vi "AxisControl.vi"(0 "String in":string, 1 "AxisBounds":T5={"Min"={"Auto"=TRUE, "Value"=0.0}, "Max"={"Auto"=TRUE, "Value"=0.0}}, 3 "ticsAndGrids":T2={"tics"={"Auto"=FALSE, "ticMin"=0.0, "ticStep"=0.0, "ticMax"=0.0, "minorDivsPerMajor"=0, "Mirror tics"=TRUE}, "Grids"={"Gridlines"=enum."No grids", "Zeroaxis"=enum."No zero axis"}}, 5 "Axis":T7="x", 9 "ShowNumbers?":bool=TRUE, 11 "ShowLabel?":bool=TRUE, 12 "Axis Label":string, 13 "Min tic value":dbl=0.001, 14 "Values":dbl[](array[numeric]), 15 "No of Tics":i32=2) -> (4 "String out":string)   [LabVIEW 2012]
uses:
  axisName.ctl
  minAndMax.ctl
  AxisScale.ctl
  ticsAndGrids.ctl
  tics.ctl
  grids.ctl
  commandArray.ctl
panel:
  out "Commands":T1
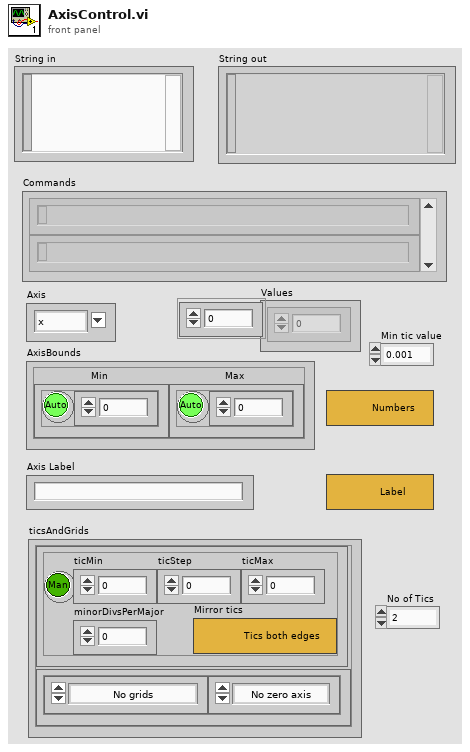
[diagram p1: front panel]
types:
  T1 = typedef "commandArray.ctl" = string[]
  T2 = typedef "ticsAndGrids.ctl" = cluster{"tics":T3, "Grids":T4}
  T3 = typedef "tics.ctl" = cluster{"Auto":bool, "ticMin":dbl, "ticStep":dbl, "ticMax":dbl, "minorDivsPerMajor":i32, "Mirror tics":bool}
  T4 = typedef "grids.ctl" = cluster{"Gridlines":enum16{"No grids", "Major grid", "Minor grid", "Major and Minor"}, "Zeroaxis":enum16{"No zero axis", "Show zero axis"}}
  T5 = typedef "minAndMax.ctl" = cluster{"Min":T6, "Max":T6}
  T6 = typedef "AxisScale.ctl" = cluster{"Auto":bool, "Value":dbl}
  T7 = typedef "axisName.ctl" = string
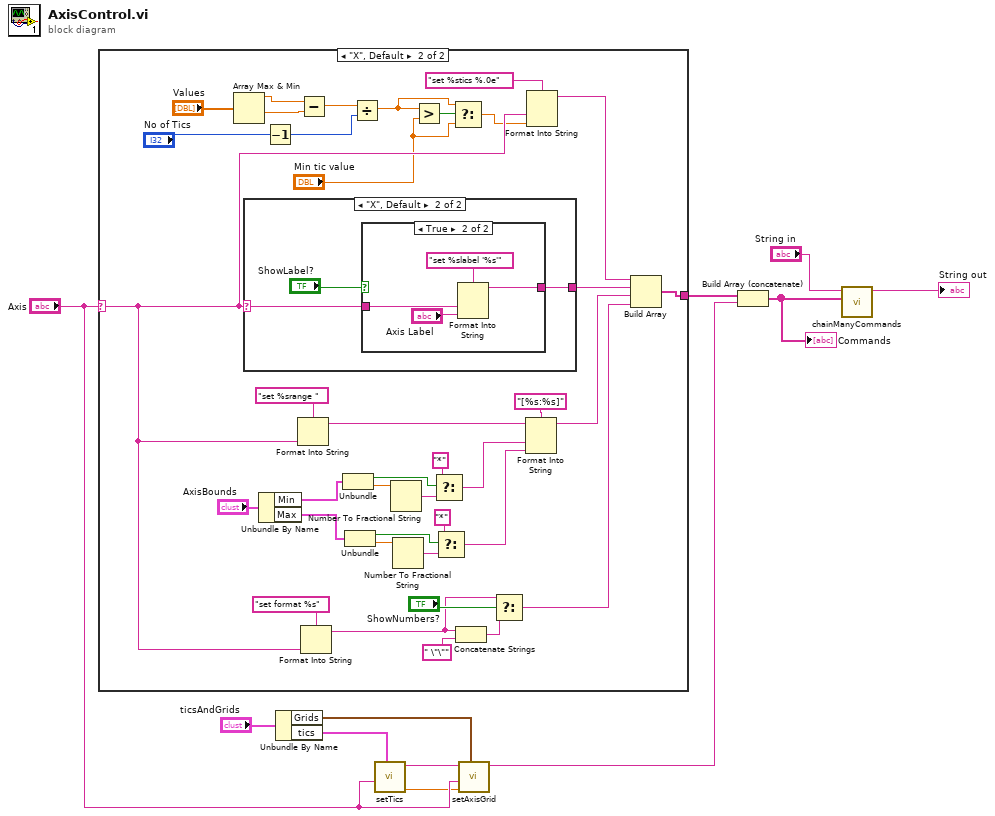
[diagram p0: block diagram]
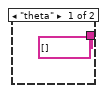
[diagram p2: hidden frame]
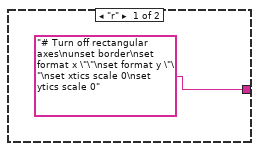
[diagram p3: hidden frame]
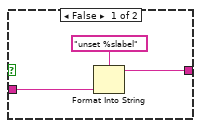
[diagram p4: hidden frame]
diagram:
  n1 = case shown="\"X\", Default" "Axis" {
    selector: "Axis" -> [_ w17]
    tunnel: [string[] [] w42] -> w7
    frame "theta" {
    }
    frame "X", Default {
      n2 = Array Max & Min(array="Values") -> (max value=w21:dbl, min value=w22:dbl)  [unwired: 2 out]
      n3 = case shown="\"X\", Default" w17 {
        selector: w17 -> [_ w52]
        tunnel: ["# Turn off rectangular axes\nunset border\nset format x \"\"\nset format y \"\"\nset xtics scale 0\nset ytics scale 0" w53] -> w40
        frame "r" {
        }
        frame "X", Default {
          n4 = case shown="True" "ShowLabel?" {
            tunnel: w52 -> [w56 w59]
            tunnel: [w55 w58] -> w53
            frame False {
              n5 = Format Into String(format string="unset %slabel", w56) -> (resulting string=w55:string)  [unwired: 2 in, 1 out]
            }
            frame True {
              n6 = Format Into String(format string="set %slabel '%s'", w59, "Axis Label") -> (resulting string=w58:string)  [unwired: 2 in, 1 out]
            }
          }
        }
      }
      n7 = Unbundle By Name("AxisBounds") -> ("Min"=w27:T6, "Max"=w26:T6)
      n8 = Decrement(x="No of Tics") -> (x-1=w25:i32)
      n9 = Format Into String(format string="set %srange ", w17) -> (resulting string=w49:string)  [unwired: 2 in, 1 out]
      n10 = Subtract(x=w21, y=w22) -> (x-y=w23:dbl)
      n11 = Format Into String(format string="set format %s", w17) -> (resulting string=w44:string)  [unwired: 2 in, 1 out]
      n12 = Unbundle(w27) -> ("Auto"=w35:bool, "Value"=w37:dbl)
      n13 = Unbundle(w26) -> ("Auto"=w33:bool, "Value"=w31:dbl)
      n14 = Divide(x=w23, y=w25) -> (x/y=w15:dbl)
      n15 = Number To Fractional String(number=w37) -> (F-format string=w38:string)  [unwired: 3 in]
      n16 = Number To Fractional String(number=w31) -> (F-format string=w30:string)  [unwired: 3 in]
      n17 = Greater?(x=w15, y="Min tic value") -> (0:w16:bool)
      n18 = Select(t="*", s=w35, f=w38) -> (s? t:f=w34:string)
      n19 = Select(t="*", s=w33, f=w30) -> (s? t:f=w29:string)
      n20 = Select(t=w15, s=w16, f="Min tic value") -> (s? t:f=w14:dbl)
      n21 = Concatenate Strings(w44, " \"\"" ("format string")) -> (w43:string)
      n22 = Select(t=w44, s="ShowNumbers?", f=w43) -> (s? t:f=w41:string)
      n23 = Format Into String(format string="[%s:%s]", initial string=w49, w34, w29) -> (resulting string=w48:string)  [unwired: 1 in, 1 out]
      n24 = Format Into String(format string="set %stics %.0e", w17, w14) -> (resulting string=w19:string)  [unwired: 2 in, 1 out]
      n25 = Build Array(w19, w40, w48, w41) -> (w42:string[])
    }
  }
  n26 = Unbundle By Name("ticsAndGrids") -> ("Grids"=w8:T4, "tics"=w9:T3)
  n27 = call "setTics.vi"("tics"=w9, "Axis"="Axis") -> ("polarGrid"=w4:dbl, "String out"=w10:string)  [unwired: 8 in]
  n28 = call "setAxisGrid.vi"("Grids"=w8, "polarGridAngle"=w4, "Axis"="Axis", "String in"=w10) -> ("String out"=w6:string)  [unwired: 7 in]
  n29 = Build Array (concatenate)(w7, w6) -> (w1:string[])
  "Commands" <- w1
  n30 = call "chainManyCommands.vi"("CommandArray"=w1, "String in in"="String in") -> ("String out"=→"String out":string)  [unwired: 9 in]
